vi "Chirp Pattern.vi"(2 "f2":dbl=0.5 format="%0.2f", 3 "f1":dbl format="%0.2f", 4 "amplitude":dbl=1.0 format="%0.2f", 5 "samples":i32=128) -> (0 "error":i32, 1 "Chirp Pattern":dbl[](array[numeric]))   [LabVIEW 2017, in "NI_AALBase.lvlib"]
doc: "Generates an array containing a chirp pattern."
uses:
  <vilib>/Analysis/NI_AALBase.lvlib
  <resource>/lvanlys.dll
panel:
  # "Chirp Pattern"
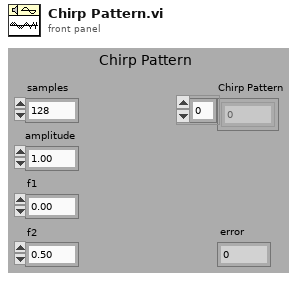
[diagram p1: front panel]
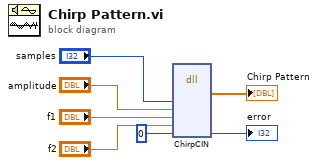
[diagram p0: block diagram]
diagram:
  n1 = dll-call lib="e:/builds/penguin/labview/branches/2017/dev/dist/resource/lvanlys.*" fn="ChirpCIN"("samples"="samples", "amplitude"="amplitude", "f1"="f1", "f2"="f2", 0) -> ("Chirp Pattern"=→"Chirp Pattern":dbl[], →"error":i32)  [unwired: 7 in, 4 out]
